vi "setUp.vi"(8 "error in (no error)":errorcluster, 11 "reference in":refnum<class "BC Major Frame.lvclass">) -> (0 "error out":errorcluster, 3 "reference out":refnum<class "BC Major Frame.lvclass">)   [LabVIEW 2016, in "BC Major Frame.lvclass"]
doc: "setUp runs prior to the test method during test execution. Use this method to initialize any object data required by your tests."
uses:
  BC Major Frame.lvclass
  <vilib>/addons/_JKI Toolkits/VI Tester/TestCase.llb/TestCase.lvclass
  Dependencies/Registry/Registry.lvclass
  D:/SVN/Products/SLSC/Multichannel 1553 Module/Software/Source Code/Driver (Windows)/Unit Tests/1553 Test/1553 Test.lvclass
  D:/Programs/National Instruments/LabVIEW 2016/vi.lib/addons/_JKI Toolkits/VI Tester/TestCase.llb/TestCase.lvclass
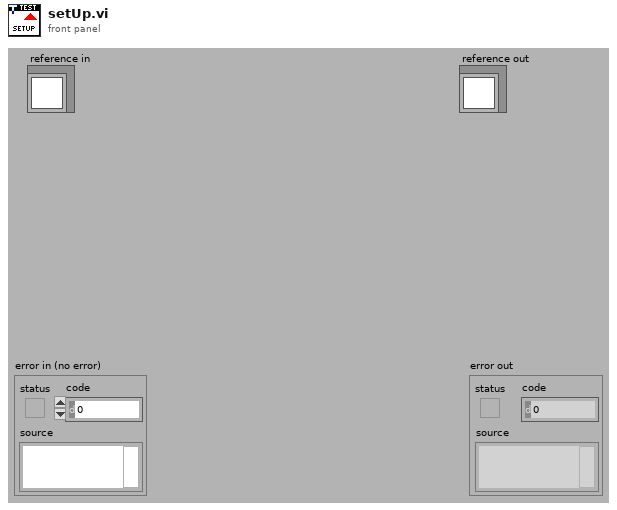
[diagram p1: front panel]
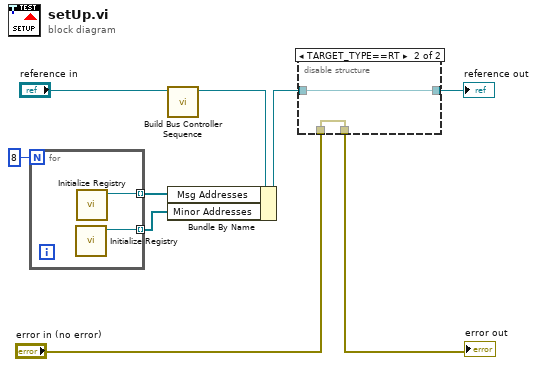
[diagram p0: block diagram]
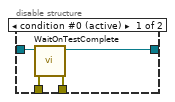
[diagram p2: hidden frame]
diagram:
  n1 = for {
    N: 8 -> [_]
    tunnel: [w11] -> w2 mode=indexing
    tunnel: [w10] -> w1 mode=indexing
    n2 = call "Initialize Registry.vi"() -> ("Registry out"=w10:refnum<class "Registry.lvclass">)  [unwired: 10 in, 1 out]
    n3 = call "Initialize Registry.vi"() -> ("Registry out"=w11:refnum<class "Registry.lvclass">)  [unwired: 10 in, 1 out]
  }
  n4 = call-dynamic "Build Bus Controller Sequence.vi"("1553 Test in"="reference in") -> ("1553 Test out"=w5:refnum<class "BC Major Frame.lvclass">)  [unwired: 9 in, 1 out]
  n5 = Bundle By Name(cluster=w5, "Msg Addresses"=w2, "Minor Addresses"=w1) -> (w4:refnum<class "BC Major Frame.lvclass">)
  n6 = disable-structure shown="TARGET_TYPE==RT" {
    disable-tunnel: "error in (no error)" -> [w15 w16]
    disable-tunnel: [w14 w16] -> w8
    disable-tunnel: [w13 w17] -> w7
    disable-tunnel: w4 -> [w12 w17]
    frame condition #0 (active) {
      n7 = call <vilib>:"WaitOnTestComplete.vi"("error in (no error)"=w15, "TestCase in"=w12) -> ("error out"=w14:errorcluster, "TestCase out"=w13:refnum<class "BC Major Frame.lvclass">)  [unwired: 8 in]
    }
    frame condition #1 {
    }
  }
  "error out" <- w8
  "reference out" <- w7
